vi "DWF MSO Query Timing.vi"(0 "Instrument Handle In":u32, 11 "Error In":errorcluster caption="Error In (no error)") -> (4 "Instrument Handle Out":u32, 6 "Sample Rate":dbl, 8 "Acquisition Time (s)":dbl, 10 "Pretrigger Time (s)":dbl, 14 "Sampling Mode":i32(ring) items=["Sample", "Peak Detect"], 15 "Error Out":errorcluster)   [LabVIEW 2015, in "DigilentWF.lvlib"]
doc: "Indicates the timing configuration of the MSO."
uses:
  <vilib>/DigilentWF/DigilentWF.lvlib
  dwf.dll
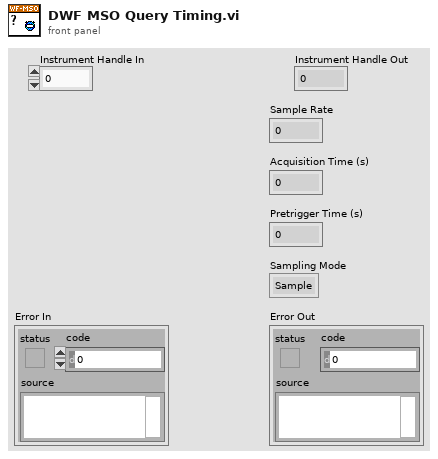
[diagram p1: front panel]
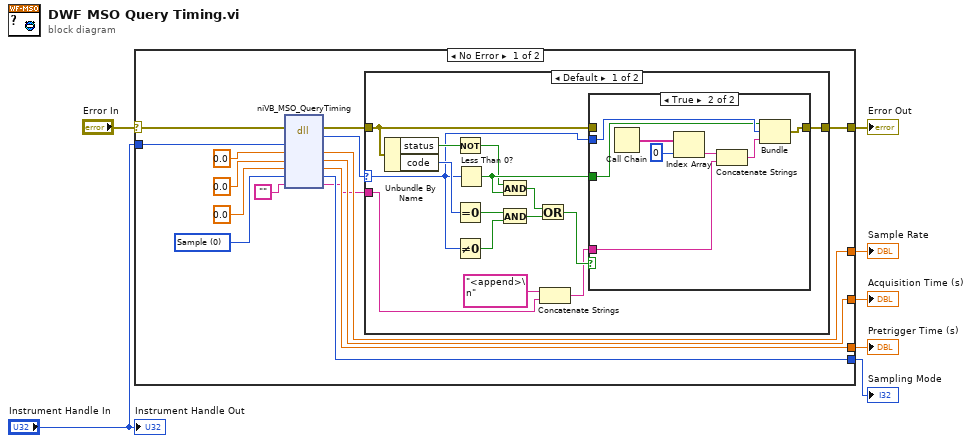
[diagram p0: block diagram]
diagram:
  n1 = case "outter_case" shown="No Error" "Error In" {
    selector: "Error In" -> [w22 w48]
    tunnel: [w19 w48] -> w6
    tunnel: "Instrument Handle In" -> [w18 _]
    tunnel: [w13 _] -> w4
    tunnel: [w12 _] -> w3
    tunnel: [w11 _] -> w2
    tunnel: [w10 _] -> w1
    frame No Error {
      w14 = 0 items=["Sample", "Peak Detect"] ("Sampling Mode")
      n2 = dll-call lib="dwf.*" fn="niVB_MSO_QueryTiming"(error in=w22, "InstrumentHandle"=w18, "SampleRate"=0.0 ("Sample Rate"), "AcquisitionTime(s)"=0.0 ("Acquisition Time (s)"), "PretriggerTime(s)"=0.0 ("Pretrigger Time (s)"), "SamplingMode"=w14, "szError"="") -> (error out=w21:errorcluster, "return type"=w20:i32, "SampleRate"=w13:dbl, "AcquisitionTime(s)"=w12:dbl, "PretriggerTime(s)"=w11:dbl, "SamplingMode"=w10:i32, "szError"=w8:string)  [unwired: 3 in, 1 out]
      n3 = case "inner_case" shown="Default" w20 {
        selector: w20 -> [w27 _]
        tunnel: w21 -> [w28 w47]
        tunnel: [w24 w47] -> w19
        tunnel: w8 -> [w23 _]
        frame Default {
          n4 = Unbundle By Name(w28) -> ("status"=w32:bool, "code"=w36:i32)
          n5 = Not(x=w32) -> (.not. x?=w35:bool)
          n6 = Equal To 0?(x=w36) -> (x = 0?=w31:bool)
          n7 = Not Equal To 0?(x=w27) -> (x != 0?=w34:bool)
          n8 = Less Than 0?(x=w27) -> (x < 0?=w37:bool)
          n9 = And(x=w35, y=w37) -> (x .and. y?=w33:bool)
          n10 = And(x=w31, y=w34) -> (x .and. y?=w30:bool)
          n11 = Or(x=w33, y=w30) -> (x .or. y?=w29:bool)
          n12 = Concatenate Strings("<append>\n" ("string"), w23) -> (w26:string)
          n13 = case shown="True" w29 {
            tunnel: [w38 w45] -> w24
            tunnel: w27 -> [_ w44]
            tunnel: w37 -> [_ w43]
            tunnel: w28 -> [w38 _]
            tunnel: w26 -> [_ w39]
            frame False {
            }
            frame True {
              n14 = Call Chain() -> (call chain=w42:string[])
              n15 = Index Array(array=w42, index=0) -> (element=w41:string)
              n16 = Concatenate Strings(w41, w39) -> (w46:string)
              n17 = Bundle(w43, "return type"=w44, w46) -> (w45:cluster{bool, "return type":i32, string})  [unwired: 1 out]
            }
          }
        }
        frame 0 {
        }
      }
    }
    frame Error {
    }
  }
  "Error Out" <- w6
  "Sample Rate" <- w4
  "Acquisition Time (s)" <- w3
  "Pretrigger Time (s)" <- w2
  "Sampling Mode" <- w1
  "Instrument Handle Out" <- "Instrument Handle In"
